vi "Read Node ID.vi"(8 "error in (no error)":errorcluster, 11 "DMA Channel Testing in":refnum<class "FPGA Addon DMA Channel Unit Tests.lvclass">) -> (0 "error out":errorcluster, 2 "Node ID":u64, 3 "DMA Channel Testing out":refnum<class "FPGA Addon DMA Channel Unit Tests.lvclass">)   [LabVIEW 2018, in "FPGA Addon DMA Channel Unit Tests.lvclass"]
uses:
  FPGA Addon DMA Channel Unit Tests.lvclass
  FPGA Addon DMA Channel Unit Tests.lvclass/FPGA Addon DMA Channel Unit Tests.ctl
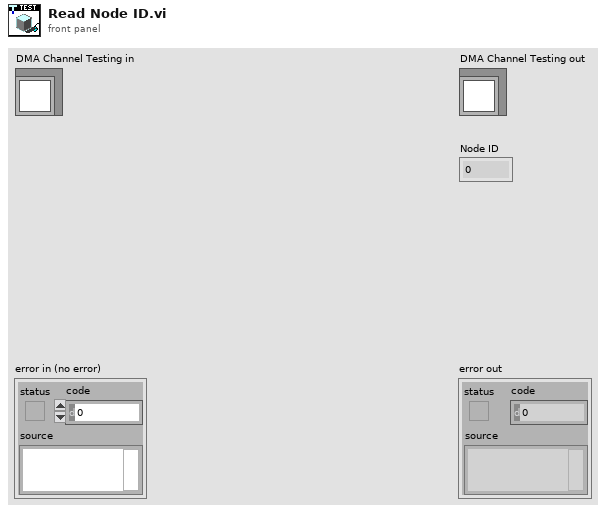
[diagram p1: front panel]
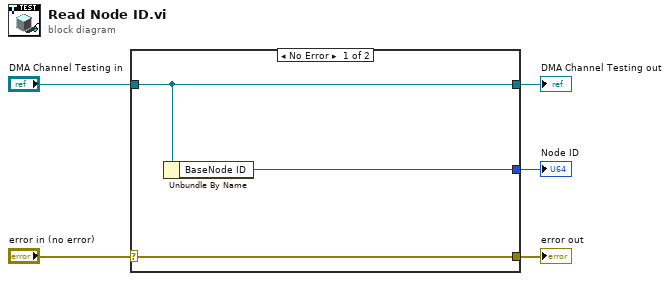
[diagram p0: block diagram]
diagram:
  n1 = case shown="No Error" "error in (no error)" {
    selector: "error in (no error)" -> [w8 w9]
    tunnel: [w8 w9] -> w4
    tunnel: [w7 w10] -> w2
    tunnel: "DMA Channel Testing in" -> [w7 w10]
    tunnel: [w6 _] -> w1
    frame No Error {
      n2 = Unbundle By Name(w7) -> ("BaseNode ID"=w6:u64)
    }
    frame Error {
    }
  }
  "error out" <- w4
  "DMA Channel Testing out" <- w2
  "Node ID" <- w1
